vi "填充.vi"(10 "初始种子":cluster{"x":u16, "y":u16}, 11 "输入数组":u8[][](array[numeric])=array106x113[11978 elements]) -> (3 "输出数组":u8[][](array[numeric]))   [LabVIEW 2014]
panel:
  out "错误输出":errorcluster
  in  "新种子":cluster{"x":u16, "y":u16}
  in  "下左边界":cluster{"x":u16, "y":u16}
  in  "下右边界":cluster{"x":u16, "y":u16}
  in  "上左边界":cluster{"x":u16, "y":u16}
  in  "空种子":cluster{"x":u16, "y":u16}
  in  "上右边界":cluster{"x":u16, "y":u16}
  # "9"
  # "27"
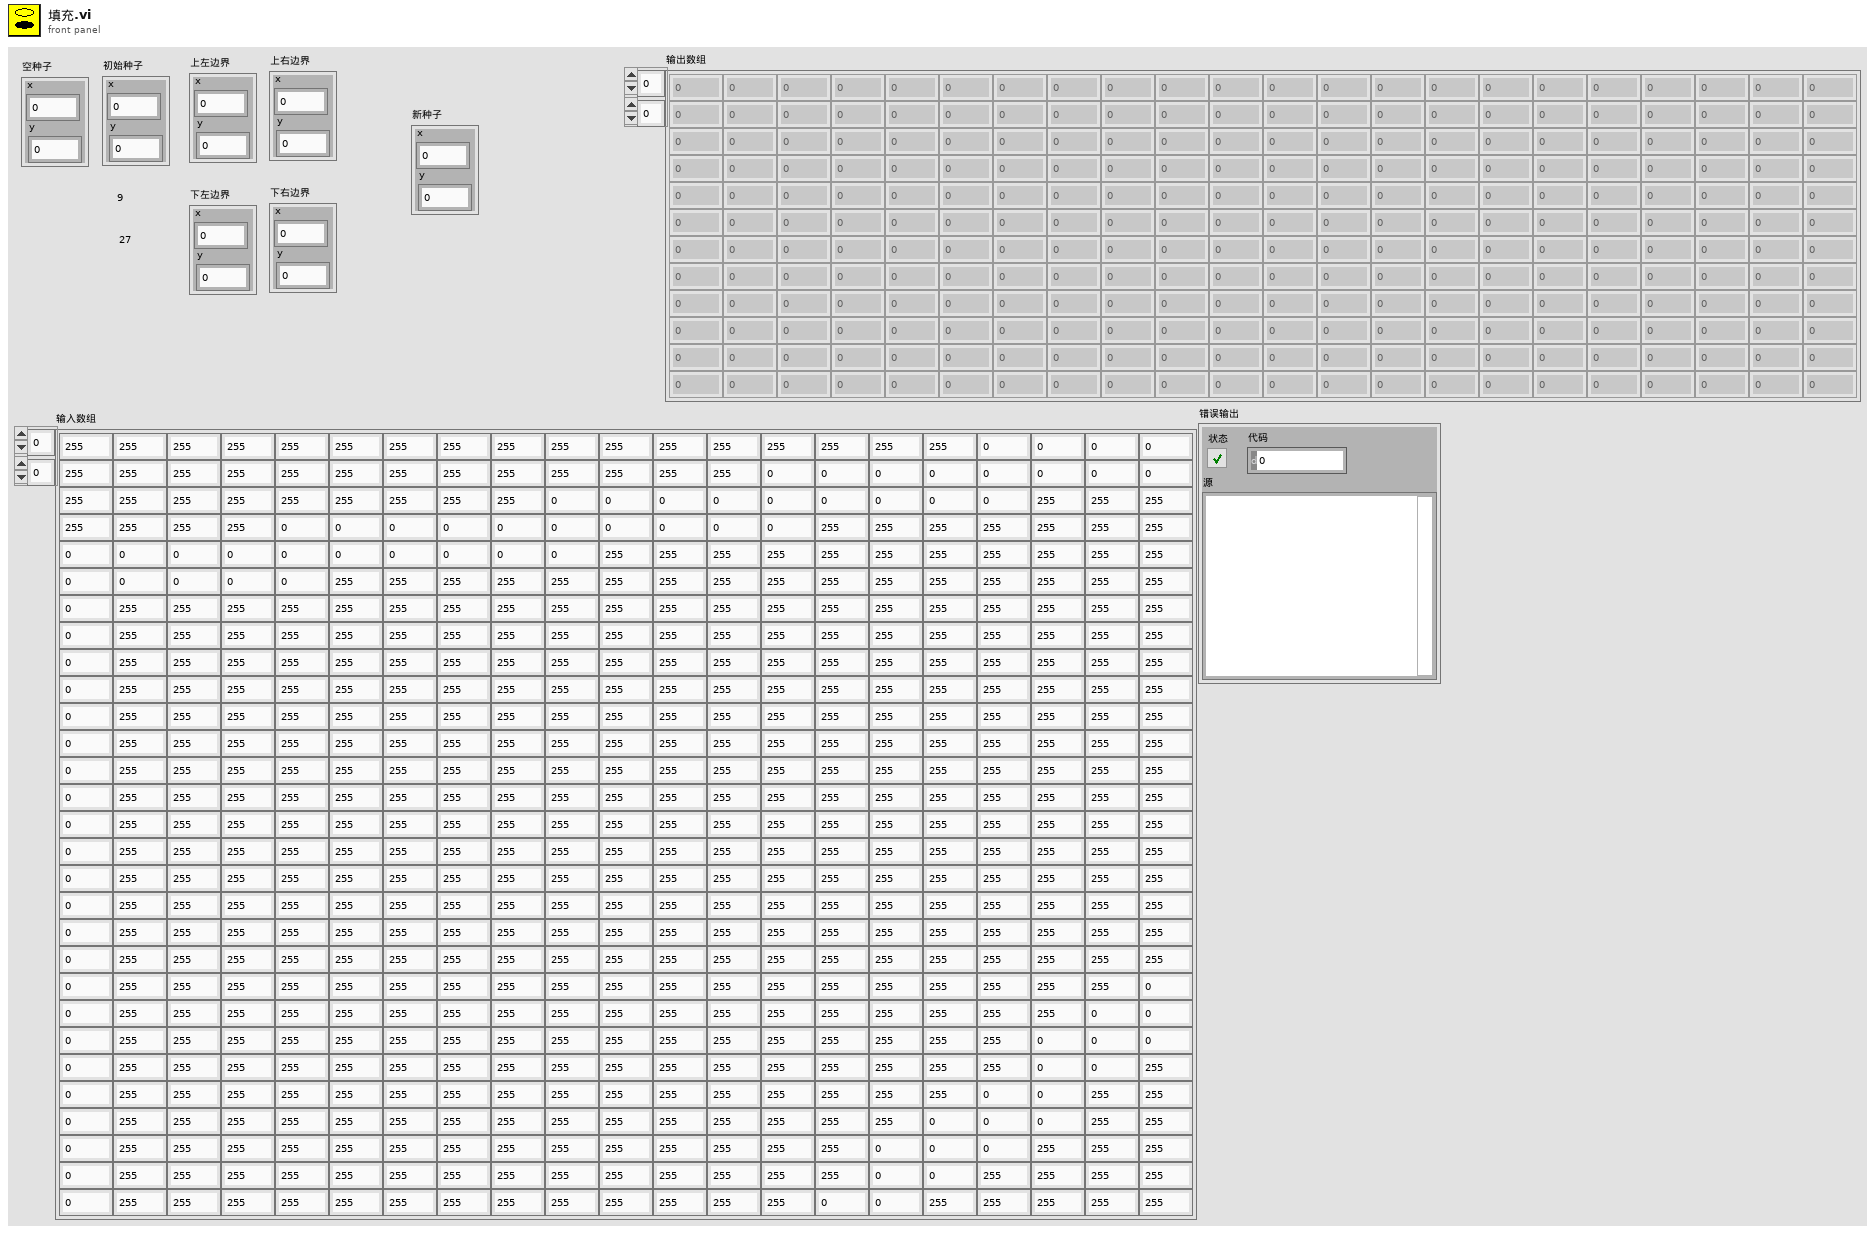
[diagram p1: front panel]
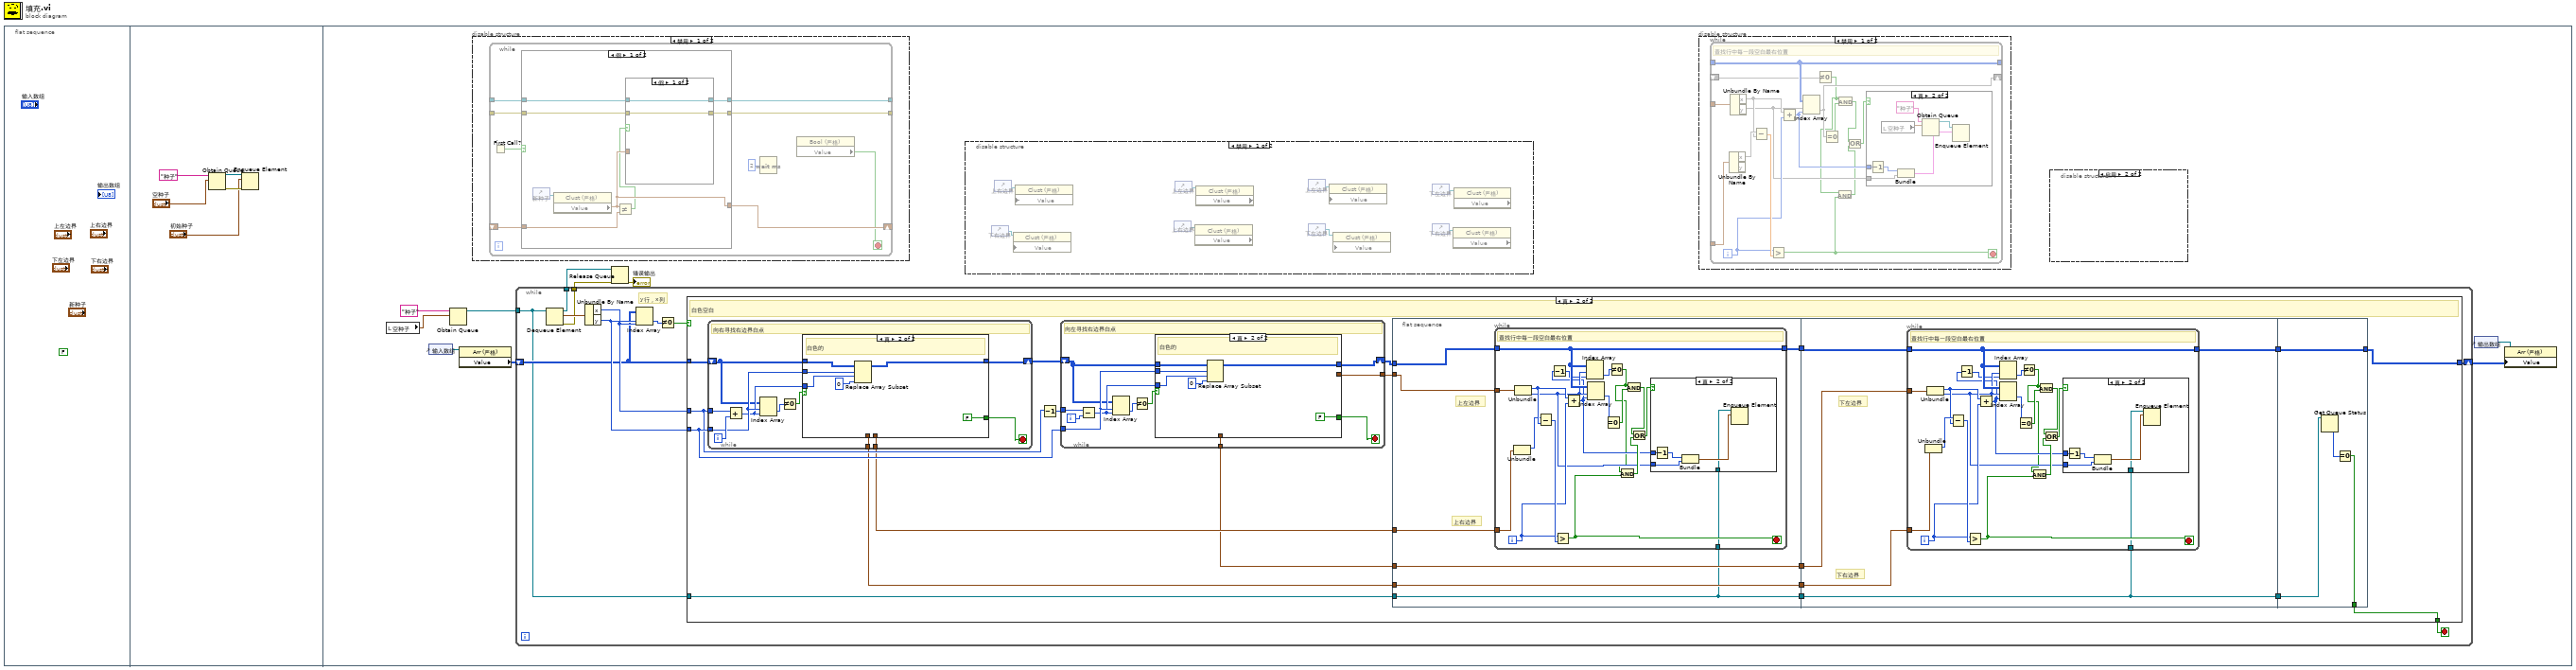
[diagram p0: block diagram]
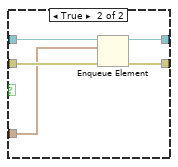
[diagram p5: hidden frame]
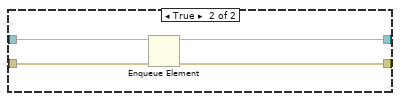
[diagram p6: hidden frame]
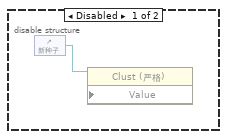
[diagram p8: hidden frame]
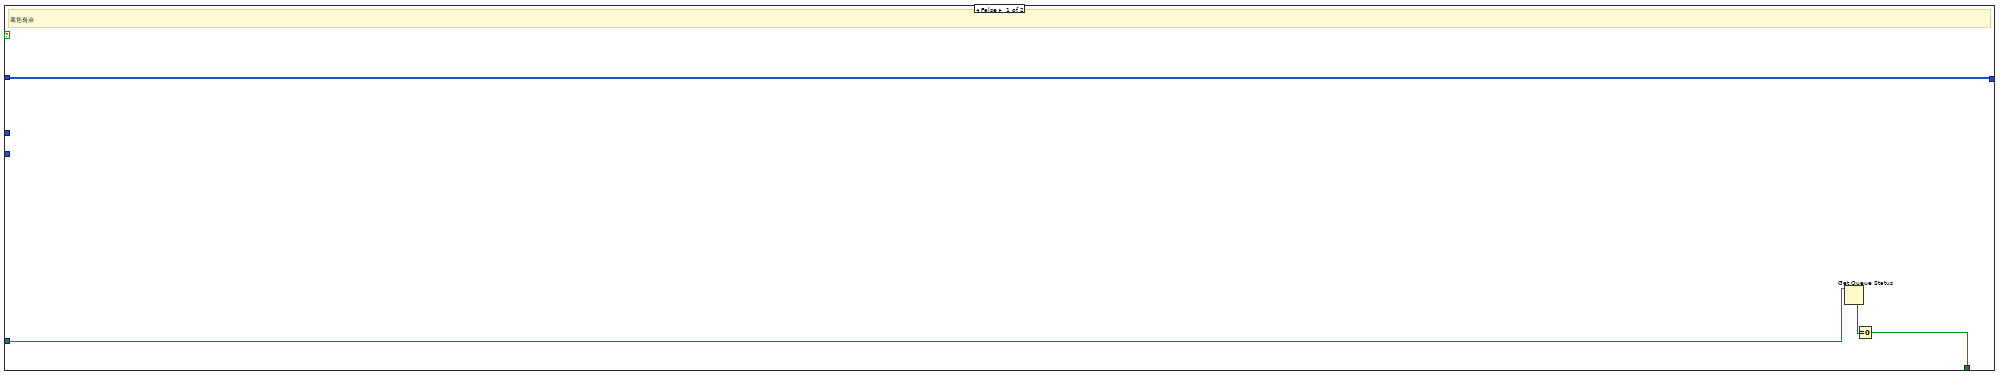
[diagram p9: hidden frame]
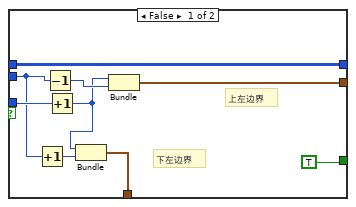
[diagram p12: hidden frame]
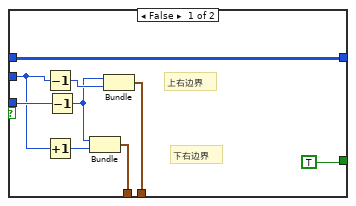
[diagram p13: hidden frame]
diagram:
  n1 = flat-sequence {
    frame #0 {
      (unwired) FALSE ("上while停")
    }
    frame #1 {
      n2 = Obtain Queue(name (unnamed)="种子" ("名称（未命名）"), element data type="空种子") -> (queue out=w4:refnum<queue>, error out=w3:errorcluster)  [unwired: 3 in, 1 out]
      n3 = Enqueue Element(queue=w4, element="初始种子", error in (no error)=w3) -> ()  [unwired: 1 in, 3 out]
    }
    frame #2 {
      n4 = local read "空种子"() -> (w13:cluster{"x":u16, "y":u16})
      n5 = control-ref of="输入数组"() -> (w8:refnum<vi>)
      n6 = Obtain Queue(name (unnamed)="种子" ("名称（未命名）"), element data type=w13) -> (queue out=w14:refnum<queue>)  [unwired: 3 in, 2 out]
      n7 = property class="Arr (严格)"(reference=w8) -> ("Value"=w7:u8[][])  [unwired: 1 in, 2 out]
      n8 = disable-structure shown="禁用" {
        frame Disabled {
          n9 = while {
            tunnel: _ -> [w56]
            tunnel: _ -> [w54]
            shift-right: [w53] -> _
            shift-left: _ -> [w52]
            tunnel: [w49] -> _
            tunnel: [w48] -> _
            stop <- w50 stop-if-true
            n10 = First Call?() -> (First Call?: T/F=w55:bool)
            n11 = case shown="假" w55 {
              tunnel: w54 -> [w61 w75]
              tunnel: w56 -> [w64 w74]
              tunnel: [w62 _] -> w53
              tunnel: w52 -> [w63 _]
              tunnel: [w60 w73] -> w49
              tunnel: [w59 w72] -> w48
              frame False {
                n12 = control-ref of="新种子"() -> (w58:refnum<vi>)
                n13 = property class="Clust (严格)"(reference=w58) -> ("Value"=w62:cluster{"x":u16, "y":u16})  [unwired: 1 in, 2 out]
                n14 = Not Equal?(x=w62, y=w63) -> (x != y?=w57:bool)
                n15 = case shown="假" w57 {
                  tunnel: w61 -> [w66 w71]
                  tunnel: w64 -> [w65 w70]
                  tunnel: w62 -> [_ w69]
                  tunnel: [w66 w68] -> w60
                  tunnel: [w65 w67] -> w59
                  frame False {
                  }
                  frame True {
                    n16 = Enqueue Element(queue=w71, element=w69, error in (no error)=w70) -> (queue out=w68:refnum<queue>, error out=w67:errorcluster)  [unwired: 1 in, 1 out]
                  }
                }
              }
              frame True {
                n17 = Enqueue Element(queue=w75, error in (no error)=w74) -> (queue out=w73:refnum<queue>, error out=w72:errorcluster)  [unwired: 2 in, 1 out]
              }
            }
            n18 = Wait (ms)(milliseconds to wait=u32 2 ("等待时间（毫秒）")) -> ()  [unwired: 1 out]
            n19 = property class="Bool (严格)"() -> ("Value"=w50:bool)  [unwired: 2 in, 2 out]
          }
        }
        frame Enabled {
        }
      }
      n20 = while {
        tunnel: w14 -> [w77]
        tunnel: [w81] -> w12
        tunnel: [w80] -> w11
        shift-right: [w78] -> w6
        shift-left: w7 -> [w79]
        stop <- w82 stop-if-true
        # "y行，x列"
        n21 = Dequeue Element(queue=w77) -> (queue out=w81:refnum<queue>, element=w83:cluster{"x":u16, "y":u16}, error out=w80:errorcluster)  [unwired: 2 in, 1 out]
        n22 = Unbundle By Name(w83) -> ("x"=w84:u16, "y"=w85:u16)
        n23 = Index Array(array=w79, index (row)=w85, index (col)=w84) -> (element=w87:u8)
        n24 = Not Equal To 0?(x=w87) -> (x != 0?=w86:bool)
        n25 = case shown="真" w86 {
          tunnel: w84 -> [_ w106]
          tunnel: w85 -> [_ w108]
          tunnel: w79 -> [w89 w110]
          tunnel: [w90 w104] -> w82
          tunnel: [w89 w101] -> w78
          tunnel: w77 -> [w88 w94]
          frame False {
            # "黑色有点"
            n26 = Get Queue Status(queue=w88) -> (# elements in queue=w91:i32)  [unwired: 2 in, 7 out]
            n27 = Equal To 0?(x=w91) -> (x = 0?=w90:bool)
          }
          frame True {
            # "白色空白"
            n28 = while {
              tunnel: w106 -> [w211]
              tunnel: w108 -> [w207]
              shift-right: [w204] -> w109
              shift-left: w110 -> [w203]
              tunnel: [w202] -> w99
              tunnel: [w201] -> w96
              i -> [w210]
              stop <- w205 stop-if-true
              # "向右寻找右边界白点"
              n29 = Add ("加")(x=w211, y=w210) -> (x+y=w206:u16)
              n30 = Index Array(array=w203, index (row)=w207, index (col)=w206) -> (element=w209:u8)
              n31 = Not Equal To 0?(x=w209) -> (x != 0?=w208:bool)
              n32 = case shown="真" w208 {
                tunnel: w203 -> [w218 w226]
                tunnel: w207 -> [w216 w225]
                tunnel: w206 -> [w219 w224]
                tunnel: [TRUE FALSE] -> w205
                tunnel: [w218 w221] -> w204
                tunnel: [w213 _] -> w202
                tunnel: [w212 _] -> w201
                frame False {
                  # "下右边界"
                  # "上右边界"
                  n33 = Decrement(x=w216) -> (x-1=w217:u16)
                  n34 = Increment(x=w216) -> (x+1=w215:u16)
                  n35 = Decrement(x=w219) -> (x-1=w214:u16)
                  n36 = Bundle(w214, w215) -> (w212:cluster{u16, u16})  [unwired: 1 in]
                  n37 = Bundle(w214, w217) -> (w213:cluster{u16, u16})  [unwired: 1 in]
                }
                frame True {
                  # "白色的"
                  n38 = Replace Array Subset(array=w226, new element=u8 0 ("新元素/子数组"), index (row)=w225, index (col)=w224) -> (w221:u8[][])
                }
              }
            }
            n39 = Decrement(x=w106) -> (x-1=w107:u16)
            n40 = while {
              tunnel: w107 -> [w185]
              tunnel: w108 -> [w182]
              shift-right: [w179] -> w105
              shift-left: w109 -> [w178]
              tunnel: [w176] -> w100
              tunnel: [w175] -> w98
              i -> [w177]
              stop <- w180 stop-if-true
              # "向左寻找右边界白点"
              n41 = Subtract ("减")(x=w185, y=w177) -> (x-y=w181:u16)
              n42 = Index Array(array=w178, index (row)=w182, index (col)=w181) -> (element=w184:u8)
              n43 = Not Equal To 0?(x=w184) -> (x != 0?=w183:bool)
              n44 = case shown="真" w183 {
                tunnel: w178 -> [w192 w200]
                tunnel: w182 -> [w190 w199]
                tunnel: w181 -> [w193 w198]
                tunnel: [TRUE FALSE] -> w180
                tunnel: [w192 w195] -> w179
                tunnel: [w187 _] -> w176
                tunnel: [w186 _] -> w175
                frame False {
                  # "下左边界"
                  # "上左边界"
                  n45 = Increment(x=w190) -> (x+1=w191:u16)
                  n46 = Decrement(x=w190) -> (x-1=w189:u16)
                  n47 = Increment(x=w193) -> (x+1=w188:u16)
                  n48 = Bundle(w188, w191) -> (w186:cluster{u16, u16})  [unwired: 1 in]
                  n49 = Bundle(w188, w189) -> (w187:cluster{u16, u16})  [unwired: 1 in]
                }
                frame True {
                  # "白色的"
                  n50 = Replace Array Subset(array=w200, new element=u8 0 ("新元素/子数组"), index (row)=w199, index (col)=w198) -> (w195:u8[][])
                }
              }
            }
            n51 = flat-sequence {
              tunnel: w105 -> [w117]
              tunnel: [w116] -> w103
              tunnel: w100 -> [w115]
              tunnel: w99 -> [w114]
              tunnel: w98 -> [w113]
              tunnel: [w113] -> w97
              tunnel: w96 -> [w112]
              tunnel: [w112] -> w95
              tunnel: w94 -> [w111]
              tunnel: [w111] -> w93
              tunnel: w103 -> [w146]
              tunnel: [w145] -> w102
              tunnel: w97 -> [w144]
              tunnel: w95 -> [w143]
              tunnel: w93 -> [w142]
              tunnel: [w142] -> w92
              tunnel: [w173] -> w104
              tunnel: [w172] -> w101
              tunnel: w102 -> [w172]
              tunnel: w92 -> [w171]
              frame #0 {
                # "上右边界"
                # "上左边界"
                n52 = while {
                  tunnel: w115 -> [w136]
                  tunnel: w114 -> [w135]
                  tunnel: w117 -> [w125]
                  tunnel: [w125] -> w116
                  tunnel: w111 -> [w118]
                  i -> [w133]
                  stop <- w129 stop-if-true
                  # "查找行中每一段空白最右位置"
                  n53 = Unbundle(w135) -> (w119:u16)  [unwired: 1 out]
                  n54 = Unbundle(w136) -> (w132:u16, w124:u16)
                  n55 = Subtract(x=w119, y=w132) -> (x-y=w134:u16)
                  n56 = Greater?(x=w133, y=w134) -> (0:w129:bool)
                  n57 = Add(x=w132, y=w133) -> (x+y=w122:i32)
                  n58 = Decrement(x=w122) -> (x-1=w123:i32)
                  n59 = Index Array(array=w125, index (row)=w124, index (col)=w123) -> (element=w121:u8)
                  n60 = Index Array(array=w125, index (row)=w124, index (col)=w122) -> (element=w131:u8)
                  n61 = Equal To 0?(x=w131) -> (x = 0?=w127:bool)
                  n62 = Not Equal To 0?(x=w121) -> (x != 0?=w120:bool)
                  n63 = And(x=w120, y=w129) -> (x .and. y?=w128:bool)
                  n64 = And(x=w120, y=w127) -> (x .and. y?=w126:bool)
                  n65 = Or(x=w126, y=w128) -> (x .or. y?=w130:bool)
                  n66 = case shown="真" w130 {
                    tunnel: w122 -> [_ w141]
                    tunnel: w124 -> [_ w139]
                    tunnel: w118 -> [_ w137]
                    frame False {
                    }
                    frame True {
                      n67 = Decrement ("减1")(x=w141) -> (x-1=w140:u16)
                      n68 = Bundle(w140, w139) -> (w138:cluster{u16, u16})  [unwired: 1 in]
                      n69 = Enqueue Element(queue=w137, element=w138) -> ()  [unwired: 2 in, 3 out]
                    }
                  }
                }
              }
              frame #1 {
                # "下左边界"
                # "下右边界"
                n70 = while {
                  tunnel: w144 -> [w165]
                  tunnel: w143 -> [w164]
                  tunnel: w146 -> [w153]
                  tunnel: [w153] -> w145
                  tunnel: w142 -> [w147]
                  i -> [w161]
                  stop <- w157 stop-if-true
                  # "查找行中每一段空白最右位置"
                  n71 = Unbundle(w164) -> (w163:u16)  [unwired: 1 out]
                  n72 = Unbundle(w165) -> (w160:u16, w152:u16)
                  n73 = Subtract(x=w163, y=w160) -> (x-y=w162:u16)
                  n74 = Greater?(x=w161, y=w162) -> (0:w157:bool)
                  n75 = Add(x=w160, y=w161) -> (x+y=w150:i32)
                  n76 = Decrement(x=w150) -> (x-1=w151:i32)
                  n77 = Index Array(array=w153, index (row)=w152, index (col)=w151) -> (element=w149:u8)
                  n78 = Index Array(array=w153, index (row)=w152, index (col)=w150) -> (element=w159:u8)
                  n79 = Equal To 0?(x=w159) -> (x = 0?=w155:bool)
                  n80 = Not Equal To 0?(x=w149) -> (x != 0?=w148:bool)
                  n81 = And(x=w148, y=w157) -> (x .and. y?=w156:bool)
                  n82 = And(x=w148, y=w155) -> (x .and. y?=w154:bool)
                  n83 = Or(x=w154, y=w156) -> (x .or. y?=w158:bool)
                  n84 = case shown="真" w158 {
                    tunnel: w150 -> [_ w170]
                    tunnel: w152 -> [_ w168]
                    tunnel: w147 -> [_ w166]
                    frame False {
                    }
                    frame True {
                      n85 = Decrement ("减1")(x=w170) -> (x-1=w169:u16)
                      n86 = Bundle(w169, w168) -> (w167:cluster{u16, u16})  [unwired: 1 in]
                      n87 = Enqueue Element(queue=w166, element=w167) -> ()  [unwired: 2 in, 3 out]
                    }
                  }
                }
              }
              frame #2 {
                n88 = Get Queue Status(queue=w171) -> (# elements in queue=w174:i32)  [unwired: 2 in, 7 out]
                n89 = Equal To 0?(x=w174) -> (x = 0?=w173:bool)
              }
            }
          }
        }
      }
      n90 = Release Queue(queue=w12, error in (no error)=w11) -> (error out=→"错误输出":errorcluster)  [unwired: 1 in, 2 out]
      n91 = disable-structure shown="禁用" {
        frame Disabled {
          n92 = control-ref of="下右边界"() -> (w18:refnum<vi>)
          n93 = control-ref of="上右边界"() -> (w19:refnum<vi>)
          n94 = property class="Clust (严格)" props=["Value"](reference=w18) -> ()  [unwired: 2 in, 2 out]
          n95 = property class="Clust (严格)" props=["Value"](reference=w19) -> ()  [unwired: 2 in, 2 out]
          n96 = control-ref of="上右边界"() -> (w23:refnum<vi>)
          n97 = control-ref of="上左边界"() -> (w22:refnum<vi>)
          n98 = property class="Clust (严格)" props=["Value"](reference=w23) -> ()  [unwired: 1 in, 3 out]
          n99 = property class="Clust (严格)" props=["Value"](reference=w22) -> ()  [unwired: 1 in, 3 out]
          n100 = control-ref of="上左边界"() -> (w21:refnum<vi>)
          n101 = control-ref of="下左边界"() -> (w20:refnum<vi>)
          n102 = property class="Clust (严格)" props=["Value"](reference=w21) -> ()  [unwired: 2 in, 2 out]
          n103 = property class="Clust (严格)" props=["Value"](reference=w20) -> ()  [unwired: 2 in, 2 out]
          n104 = control-ref of="下右边界"() -> (w16:refnum<vi>)
          n105 = control-ref of="下左边界"() -> (w17:refnum<vi>)
          n106 = property class="Clust (严格)" props=["Value"](reference=w16) -> ()  [unwired: 1 in, 3 out]
          n107 = property class="Clust (严格)" props=["Value"](reference=w17) -> ()  [unwired: 1 in, 3 out]
        }
        frame Enabled {
        }
      }
      n108 = disable-structure shown="禁用" {
        frame Disabled {
          n109 = while {
            tunnel: _ -> [w40]
            tunnel: _ -> [w39]
            tunnel: _ -> [w34]
            tunnel: [w34] -> _
            shift-right: [w32] -> _
            shift-left: _ -> [w33]
            i -> [w36]
            stop <- w25 stop-if-true
            # "查找行中每一段空白最右位置"
            n110 = Unbundle By Name(w39) -> ("x"=w38)  [unwired: 1 out]
            n111 = Unbundle By Name(w40) -> ("x"=w35, "y"=w30)
            n112 = Subtract(x=w38, y=w35) -> (x-y=w37:dbl)
            n113 = Greater?(x=w36, y=w37) -> (0:w25:bool)
            n114 = Add(x=w35, y=w36) -> (x+y=w31:i32)
            n115 = Index Array(array=w34, index (row)=w30, index (col)=w31) -> (element=w32)
            n116 = Not Equal To 0?(x=w33) -> (x != 0?=w26:bool)
            n117 = Equal To 0?(x=w32) -> (x = 0?=w29:bool)
            n118 = And(x=w26, y=w25) -> (x .and. y?=w24:bool)
            n119 = And(x=w26, y=w29) -> (x .and. y?=w27:bool)
            n120 = Or(x=w27, y=w24) -> (x .or. y?=w28:bool)
            n121 = case shown="真" w28 {
              tunnel: w31 -> [_ w47]
              tunnel: w30 -> [_ w45]
              frame False {
              }
              frame True {
                n122 = Decrement(x=w47) -> (x-1=w46:i32)
                n123 = local read "空种子"() -> (w43:cluster{"x":u16, "y":u16})
                n124 = Bundle(w46, "y"=w45) -> (w41:cluster{i32, "y":void})  [unwired: 1 in]
                n125 = Obtain Queue(name (unnamed)="种子" ("名称（未命名）"), element data type=w43) -> (queue out=w44:refnum<queue>)  [unwired: 3 in, 2 out]
                n126 = Enqueue Element(queue=w44, element=w41) -> ()  [unwired: 2 in, 3 out]
              }
            }
          }
        }
        frame Enabled {
        }
      }
      n127 = disable-structure shown="启用" {
        frame Disabled {
          n128 = control-ref of="新种子"() -> (w76:refnum<vi>)
          n129 = property class="Clust (严格)" props=["Value"](reference=w76) -> ()  [unwired: 2 in, 2 out]
        }
        frame Enabled {
        }
      }
      n130 = control-ref of="输出数组"() -> (w9:refnum<vi>)
      n131 = property class="Arr (严格)"(reference=w9, "Value"=w6) -> ()  [unwired: 1 in, 2 out]
    }
  }
